vi "Sort Array and Reorder Array Example 01.vi"() -> ()   [LabVIEW 2019]
uses:
  user.lib/_OpenG.lib/array/array.llb/Sort 1D Array (U8)__ogtk.vi
  user.lib/_OpenG.lib/array/array.llb/Reorder 1D Array2 (String)__ogtk.vi
panel:
  out "Names Sorted by Grades":string[](array[string])
  in  "Corresponding Grades":u8[](array[numeric])=[87, 34, 16, 23, 98, 67, 56, 24, 73]
  in  "Unsorted Names":string[](array[string])=["Frank", "Alice", "Raphael", "Walter", "Beatrice", "Harry", "Diane", "Cleo", "Lester"]
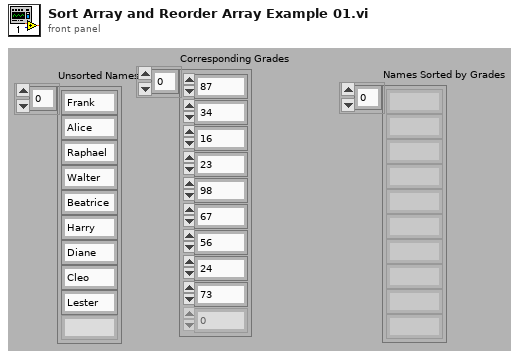
[diagram p1: front panel]
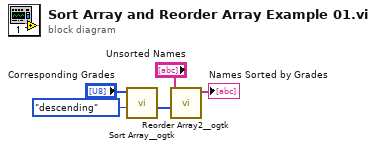
[diagram p0: block diagram]
diagram:
  n1 = call-poly "Sort Array__ogtk.vi"("Order"=enum16{"ascending", "descending"}."descending", "Array in"="Corresponding Grades") -> ("Sorted Pointers"=w2:i32[])  [unwired: 8 in, 1 out]
  n2 = call-poly "Reorder Array2__ogtk.vi"("indices"=w2, "array"="Unsorted Names") -> ("reordered array"=→"Names Sorted by Grades":string[])  [unwired: 9 in]
